vi "Write Binary Configuration.vi"(7 "Type":T1, 8 "error in (no error)":errorcluster, 9 "Value":variant, 10 "Name":string, 11 "TransientConfiguration in":refnum<class "TransientConfiguration.lvclass">) -> (0 "error out":errorcluster, 3 "TransientConfiguration out":refnum<class "TransientConfiguration.lvclass">)   [LabVIEW 2020, in "TransientConfiguration.lvclass"]
uses:
  <vilib>/gpm_packages/@cs/Configuration/Source/TransientConfiguration/TransientConfiguration.lvclass
  <vilib>/Utility/Data Type/Type Definitions/Data Type.ctl
  <vilib>/gpm_packages/@cs/Configuration/Source/TransientConfiguration/TransientConfiguration.lvclass/TransientConfiguration.ctl
  <vilib>/Utility/Data Type/NI_Data Type.lvlib
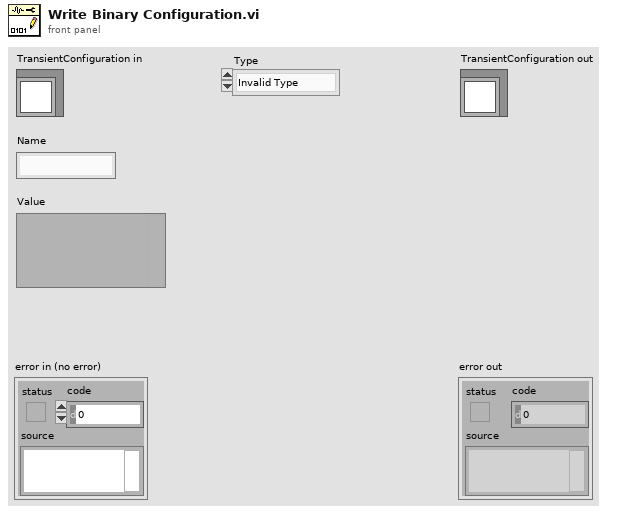
[diagram p1: front panel]
types:
  T1 = typedef "NI_Data Type.lvlib/Data Type.ctl" = enum8{"Invalid Type", "Void", "I8", "I16", "I32", "I64", "U8", "U16", "U32", "U64", "Single Float", "Double Float", "Extended Float", "Single Complex", "Double Complex", "Extended Complex", "Enum U8", "Enum U16", "Enum U32", "Enum U64", "Single Float With Unit", "Double Float With Unit", "Extended Float With Unit", "Single Complex with Unit", "Double Complex with Unit", "Extended Complex with Unit", "Boolean", "String", "Path", "Picture", "Tag", "Array", "Cluster", "Variant", "LV Variant", "Waveform", "Timestamp", "Digital Waveform", "Digital Data", "ExpressData", "Refnum", "External Data", "VI", "Poly VI", "LabVIEW Class Instance", "Fixed Point", "Set Collection", "Map Collection"}
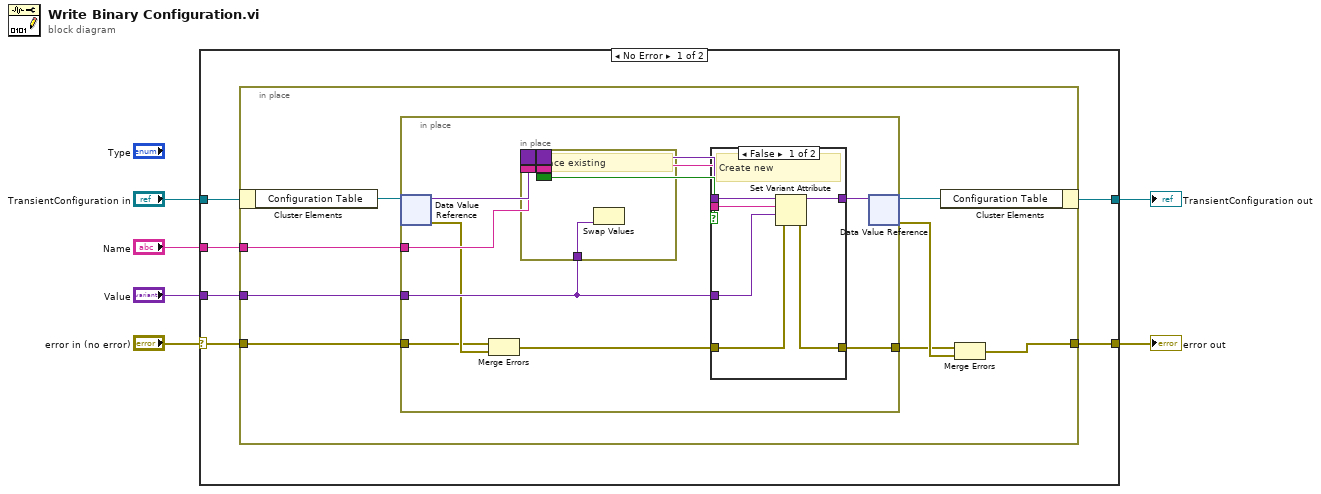
[diagram p0: block diagram]
diagram:
  n1 = case shown="No Error" "error in (no error)" {
    selector: "error in (no error)" -> [w7 w45]
    tunnel: "TransientConfiguration in" -> [w12 w44]
    tunnel: [w11 w44] -> w5
    tunnel: "Name" -> [w10 _]
    tunnel: "Value" -> [w9 _]
    tunnel: [w8 w45] -> w1
    frame No Error {
      n2 = in-place {
        in-place-border: w10 -> [w18]
        in-place-border: w9 -> [w17]
        in-place-border: [w14] -> w8
        in-place-border: w7 -> [w13]
        n3 = in-place-cluster #1(w12) -> ("Configuration Table"=w20:refnum<data-value>)
        n4 = in-place {
          in-place-border: w18 -> [w30]
          in-place-border: w17 -> [w25]
          in-place-border: [w23] -> w15
          in-place-border: w13 -> [w21]
          n5 = in-place-dvr #2(w20) -> (w31:variant, w24:errorcluster)
          n6 = Merge Errors(w21, w24) -> (w22:errorcluster)
          n7 = in-place {
            border: w31 -> [_]
            border: w30 -> [_]
            border: [_] -> w28
            border: [_] -> w26
            border: [_] -> w29
            in-place-border: w25 -> [w40]
            # "Replace existing"
            n8 = Swap Values(12:w42, 13:w43, 14:w40) -> (1:w41:variant)  [unwired: 1 out]
          }
          n9 = case shown="False" w29 {
            tunnel: w28 -> [w37 w39]
            tunnel: [w36 w39] -> w27
            tunnel: w26 -> [w35 _]
            tunnel: w25 -> [w34 _]
            tunnel: w22 -> [w33 w38]
            tunnel: [w32 w38] -> w23
            frame False {
              # "Create new"
              n10 = Set Variant Attribute(Variant=w37, name=w35, value=w34, error in=w33) -> (Variant out=w36:variant, error out=w32:errorcluster)  [unwired: 1 out]
            }
            frame True {
              # "Replaced"
            }
          }
          n11 = in-place-dvr #2(w27) -> (w19:refnum<data-value>, w16:errorcluster)
        }
        n12 = in-place-cluster #1("Configuration Table"=w19) -> (w11:refnum<class "TransientConfiguration.lvclass">)
        n13 = Merge Errors(w15, w16) -> (w14:errorcluster)
      }
    }
    frame Error {
    }
  }
  "error out" <- w1
  "TransientConfiguration out" <- w5
